vi "degree test.vi"(9 "x":dbl, 10 "y":dbl) -> (1 "red encoder":dbl, 2 "blue encoder":dbl)   [LabVIEW 2020]
panel:
  out "?":bool
  out "red angle":dbl
  out "Blue angle":dbl
  # "Valid x and y"
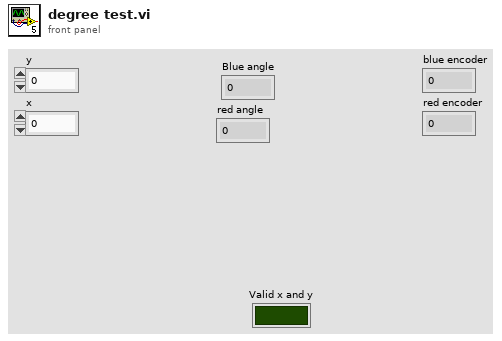
[diagram p1: front panel]
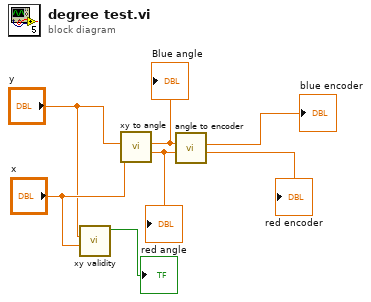
[diagram p0: block diagram]
diagram:
  n1 = call "xy validity.vi"("x input"="x", "y input"="y") -> ("Validity"=→"?":bool)  [unwired: 9 in]
  n2 = call "xy to angle.vi"("x"="x", "y"="y") -> ("red angle"=w2:dbl, "Blue angle"=w1:dbl)  [unwired: 8 in]
  "Blue angle" <- w1
  "red angle" <- w2
  n3 = call "angle to encoder.vi"("red angle"=w2, "blue angle"=w1) -> ("red encoder"=→"red encoder":dbl, "blue encoder"=→"blue encoder":dbl)  [unwired: 8 in]
